vi "Stop Core.vi"(10 "final error code":i32, 11 "Nested in":refnum<class "UI_CAFÉ_USD_ES.lvclass">) -> (3 "Nested out":refnum<class "UI_CAFÉ_USD_ES.lvclass">)   [LabVIEW 2019, in "UI_CAFÉ_USD_ES.lvlib" / "UI_CAFÉ_USD_ES.lvclass"]
doc: "(<B>Filename</B>: Actor Framework.lvlib:Actor.lvclass:Stop Core.vi)\n\nDefines what the actor does before it stops. Use the <B>final error code</B> input to determine whether the actor shut down in response to an error.\n\nBy default, this method does nothing. A descendant class may override it to define behavior, such as shutting down any processes the actor initiated in its override of the Actor Core method."
uses:
  <vilib>/ActorFramework/Actor/Actor.lvclass
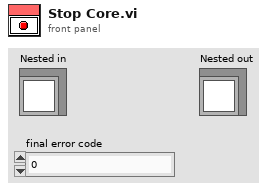
[diagram p1: front panel]
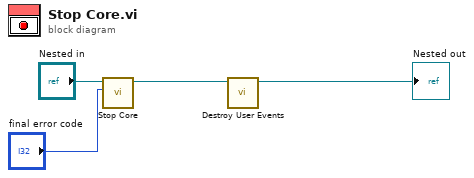
[diagram p0: block diagram]
diagram:
  n1 = call-parent "Stop Core.vi"("final error code"="final error code", "Actor in"="Nested in") -> ("Actor out"=w2:refnum<class "UI_CAFÉ_USD_ES.lvclass">)  [unwired: 9 in]
  n2 = call "Destroy User Events.vi"("UI Template in"=w2) -> ("UI Template out"=→"Nested out":refnum<class "UI_CAFÉ_USD_ES.lvclass">)  [unwired: 10 in]
